vi "append log entry.vi"(5 "Force Archive? (f)":bool, 7 "error in (no error)":errorcluster, 8 "Username (\"\")":string, 9 "Module Name (\"\")":string, 10 "Error Type (Information)":T1) -> (0 "error out":errorcluster)   [LabVIEW 2011]
uses:
  errorlog types.ctl
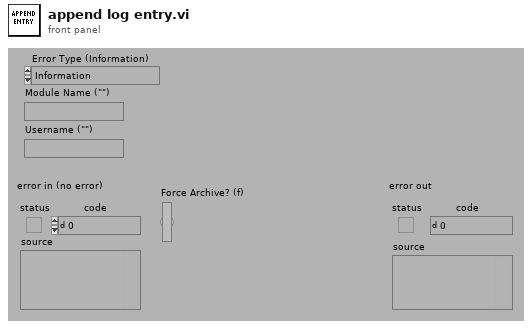
[diagram p1: front panel]
types:
  T1 = typedef "errorlog types.ctl" = enum16{"Information", "Warning", "Error"}
  T2 = enum16{"open", "replace", "create", "open or create", "replace or create", "replace or create with confirmation"}
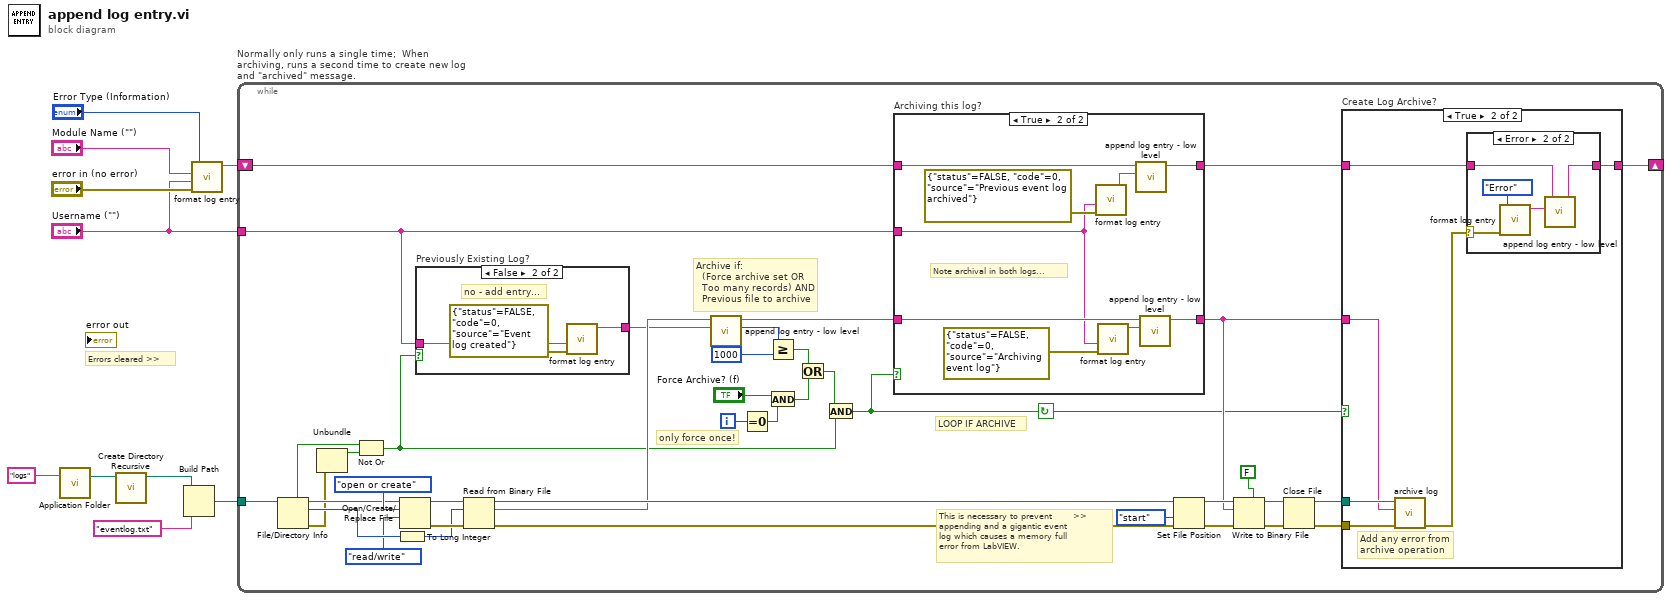
[diagram p0: block diagram]
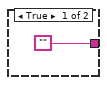
[diagram p2: hidden frame]
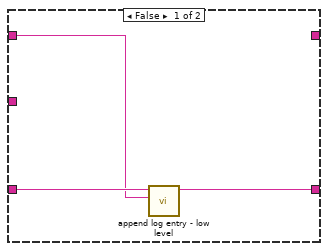
[diagram p5: hidden frame]
diagram:
  # "Errors cleared >>"
  n1 = call "Application Folder.vi"("Relative Path (\"\" - Folder)"="logs" ("name or relative path")) -> ("Application Folder"=w2:path)  [unwired: 2 in]
  n2 = call <vilib>:"Create Directory Recursive.vi"("directory"=w2) -> ("directory copy"=w4:path)  [unwired: 2 in, 4 out]
  n3 = Build Path(base path=w4, name or relative path="eventlog.txt") -> (appended path=w3:path)
  n4 = call "format log entry.vi"("error in (no error)"="error in (no error)", "Username (\"\")"="Username (\"\")", "Module Name (\"\")"="Module Name (\"\")", "Error Type (Information)"="Error Type (Information)") -> ("Error Record"=w9:string)  [unwired: 3 out]
  n5 = while "Normally only runs a single time;  When archiving, runs a second time to create new log and \"archived\" message." {
    tunnel: w3 -> [w18]
    shift-right: [w11] -> _
    shift-left: w9 -> [w20]
    tunnel: "Username (\"\")" -> [w23]
    i -> [w13]
    stop <- w19 continue-if-true
    # "LOOP IF ARCHIVE"
    # "Archive if:\n  (Force archive set OR\n  Too many records) AND\n  Previous file to archive"
    # "This is necessary to prevent       >>\nappending and a gigantic event\nlog which causes a memory full\nerror from LabVIEW."
    # "only force once!"
    n6 = File/Directory Info(path=w18) -> (path out=w43:path, directory=w33:bool, size=w42:i64, error out=w34:errorcluster)  [unwired: 1 in, 3 out]
    n7 = Unbundle(w34) -> ("status"=w32:bool)  [unwired: 2 out]
    n8 = Not Or(1:w32, 2:w33) -> (0:w21:bool)
    n9 = To Long Integer(number=w42) -> (32bit integer=w28:i32)
    n10 = Open/Create/Replace File(file path (use dialog)=w43, operation (0:open)=T2."open or create", access (0:read/write)=enum16{"read/write", "read-only", "write-only"}."read/write") -> (refnum out=w30:refnum<file>, error out=w29:errorcluster)  [unwired: 1 in, 3 out]
    n11 = case "Previously Existing Log?" shown="False" w21 {
      tunnel: ["" w51] -> w24
      tunnel: w23 -> [_ w52]
      frame True {
      }
      frame False {
        # "no - add entry..."
        n12 = call "format log entry.vi"("error in (no error)"=errorcluster {"status"=FALSE, "code"=0, "source"="Event log created"}, "Username (\"\")"=w52) -> ("Error Record"=w51:string)  [unwired: 2 in, 3 out]
      }
    }
    n13 = Read from Binary File(8:w29, 10:w28, 11:w30) -> (0:w26:errorcluster, 2:w25:string, 3:w27:refnum<file>)  [unwired: 4 out]
    n14 = call "append log entry - low level.vi"("Record to Add (\"\")"=w24, "Current Log Contents (\"\")"=w25) -> ("Records"=w49:i32, "New Log Contents"=w46:string)  [unwired: 1 in, 3 out]
    n15 = Equal To 0?(x=w13) -> (x = 0?=w15:bool)
    n16 = Greater Or Equal?(x=w49, y=1000) -> (x >= y?=w47:bool)
    n17 = And(x="Force Archive? (f)", y=w15) -> (x .and. y?=w14:bool)
    n18 = Or(x=w47, y=w14) -> (x .or. y?=w22:bool)
    n19 = And(x=w22, y=w21) -> (x .and. y?=w19:bool)
    n20 = case "Archiving this log?" shown="True" w19 {
      tunnel: w46 -> [w69 w76]
      tunnel: [w68 w74] -> w31
      tunnel: [_ w72] -> w12
      tunnel: w23 -> [_ w73]
      tunnel: w20 -> [w67 w71]
      frame False {
        n21 = call "append log entry - low level.vi"("Record to Add (\"\")"=w67, "Current Log Contents (\"\")"=w69) -> ("New Log Contents"=w68:string)  [unwired: 1 in, 4 out]
      }
      frame True {
        # "Note archival in both logs..."
        n22 = call "format log entry.vi"("error in (no error)"=errorcluster {"status"=FALSE, "code"=0, "source"="Previous event log archived"}, "Username (\"\")"=w73) -> ("Error Record"=w70:string)  [unwired: 2 in, 3 out]
        n23 = call "format log entry.vi"("error in (no error)"=errorcluster {"status"=FALSE, "code"=0, "source"="Archiving event log"}, "Username (\"\")"=w73) -> ("Error Record"=w77:string)  [unwired: 2 in, 3 out]
        n24 = call "append log entry - low level.vi"("Record to Add (\"\")"=w70, "Current Log Contents (\"\")"=w71) -> ("New Log Contents"=w72:string)  [unwired: 1 in, 4 out]
        n25 = call "append log entry - low level.vi"("Record to Add (\"\")"=w77, "Current Log Contents (\"\")"=w76) -> ("New Log Contents"=w74:string)  [unwired: 1 in, 4 out]
      }
    }
    n26 = Set File Position(refnum=w27, from (0:start)=enum16{"start", "end", "current"}."start", error in=w26) -> (refnum out=w37:refnum<file>, error out=w38:errorcluster)  [unwired: 1 out]
    n27 = Write to Binary File(file (use dialog)=w37, data=w31, error in=w38, 5:FALSE) -> (refnum out=w41:refnum<file>, error out=w40:errorcluster)  [unwired: 3 out]
    n28 = Close File(refnum=w41, error in=w40) -> (path=w17:path, error out=w45:errorcluster)
    n29 = case "Create Log Archive?" shown="True" w19 {
      tunnel: w45 -> [_ w60]
      tunnel: w17 -> [_ w59]
      tunnel: w31 -> [_ w58]
      tunnel: w12 -> [w54 w56]
      tunnel: [w54 w55] -> w11
      frame False {
      }
      frame True {
        # "Add any error from\narchive operation"
        n30 = call "archive log.vi"("error in (no error)"=w60, "Flat Log (\"\")"=w58, "Log Path (empty)"=w59) -> ("error out"=w57:errorcluster)  [unwired: 4 out]
        n31 = case shown="Error" w57 {
          selector: w57 -> [_ w62]
          tunnel: w56 -> [w61 w64]
          tunnel: [w61 w63] -> w55
          frame No Error {
          }
          frame Error {
            n32 = call "format log entry.vi"("error in (no error)"=w62, "Error Type (Information)"=errorlog_types."Error") -> ("Error Record"=w66:string)  [unwired: 2 in, 3 out]
            n33 = call "append log entry - low level.vi"("Record to Add (\"\")"=w66, "Current Log Contents (\"\")"=w64) -> ("New Log Contents"=w63:string)  [unwired: 1 in, 4 out]
          }
        }
      }
    }
  }
